vi "Run Framework Configuration.vi"(7 "framework options":T13={"FIFO Options"={"Infinite Timeouts"=FALSE}, "Thread Options"={"Show FP On Call"=TRUE, "Close FP After Call"=TRUE, "Allow Debugging"=FALSE, "Restart On Error"=FALSE}, "Plugin Options"={"Default Components"=TRUE}, "Performance Options"={"Measure Period"=TRUE, "Measure Rx/Tx Duration"=TRUE}}, 9 "target frequency":u32 format="%.0pHz", 10 "components directory":path, 11 "dsf configuration file path":path=path "C:/Users/Admin/Desktop/test.dsf") -> ()   [LabVIEW 2017, in "DSF Core.lvlib"]
uses:
  DSF Core.lvlib
  Classes/Framework/Framework Options.ctl
  Typedefs/DSF FIFO Options.ctl
  Classes/Thread/DSF Thread Options.ctl
  Typedefs/DSF Plugin Options.ctl
  Typedefs/DSF Performance Options.ctl
  Typedefs/DSF Engine Framework Configuration.ctl
  Typedefs/DSF Engine Plugin Configuration.ctl
  Typedefs/DSF Timing Info.ctl
  Typedefs/DSF Engine Plugin Thread Configuration.ctl
  Typedefs/DSF Settings Info.ctl
  Typedefs/DSF Engine Transfer Group Configuration.ctl
  Typedefs/DSF Direction.ctl
  Typedefs/DSF Engine Transfer Configuration.ctl
  Typedefs/DSF Byte Order.ctl
  Typedefs/DSF Engine Channel Configuration.ctl
  Typedefs/DSF Data Type.ctl
  Typedefs/DSF Timeout Behavior.ctl
  <vilib>/NI/Memory Manager/Classes/Pointer/Pointer.lvclass
  <vilib>/NI/Memory Manager/Classes/Pointer/Pointer.lvclass/Pointer.ctl
  <vilib>/Platform/TimedLoop/XDataNode/timing_clust.ctl
  <vilib>/Platform/TimedLoop/XDataNode/nitl_modes.ctl
  <vilib>/Platform/TimedLoop/XDataNode/wakeup.ctl
  <vilib>/NI/Memory Manager/Classes/Pointer/Write U32.vi
  <vilib>/NI/Memory Manager/Classes/Pointer/Read U32.vi
  <vilib>/NI/Memory Manager/Classes/Pointer/Read Bool.vi
  <vilib>/NI/Memory Manager/Classes/Pointer/Write Bool.vi
  <vilib>/NI/Memory Manager/Classes/Pointer/Set Address.vi
  <vilib>/NI/Memory Manager/Classes/Pointer/Set Size.vi
  <vilib>/NI/Memory Manager/Classes/Pointer/Set Internal.vi
  <vilib>/NI/Memory Manager/Classes/Pointer/Check Null Pointer.vi
  <vilib>/NI/Memory Manager/Classes/Pointer/Clear (No Check).vi
  <vilib>/NI/Memory Manager/Classes/Pointer/Check Length.vi
  <vilib>/NI/Memory Manager/Classes/Pointer/Write (No Check).vi
  <vilib>/NI/Memory Manager/Classes/Pointer/Write (No Check) U32.vi
  <vilib>/NI/Memory Manager/Classes/Pointer/Check Move.vi
  <vilib>/NI/Memory Manager/Classes/Pointer/Read (No Check).vi
  <vilib>/NI/Memory Manager/Classes/Pointer/Read (No Check) U32.vi
  <vilib>/NI/Memory Manager/Classes/Pointer/Read (No Check) Bool.vi
  <vilib>/NI/Memory Manager/Classes/Pointer/Write (No Check) Bool.vi
  <vilib>/NI/Memory Manager/Classes/Pointer/Get Internal.vi
  <vilib>/NI/Memory Manager/Classes/Pointer/Errors.vi
  <vilib>/NI/Memory Manager/Classes/Pointer/Zone.vi
  <vilib>/NI/Memory Manager/Classes/Pointer/Null Pointer.vi
  <vilib>/NI/Memory Manager/Classes/Pointer/Check Bounds (Pointer).vi
  <vilib>/NI/Memory Manager/Classes/Pointer/Check Count.vi
  <vilib>/NI/Memory Manager/Classes/Pointer/Check Bounds (Power of 2).vi
  <vilib>/NI/Memory Manager/Classes/Pointer/Create Error.vi
  <vilib>/NI/Memory Manager/Classes/Pointer/Out of Bounds.vi
  <vilib>/NI/Memory Manager/Classes/Pointer/Check Bounds.vi
  <vilib>/NI/Memory Manager/Constants/Constants.vi
  <vilib>/NI/Memory Manager/Constants/Library Name.vi
  <vilib>/NI/Memory Manager/Classes/Pointer/Pointer Error Info.vi
  <vilib>/NI/Memory Manager/Constants/Pointer Class Name.vi
  <vilib>/NI/Memory Manager/Classes/Pointer/Write Pointer Size to Error.vi
  <vilib>/NI/Memory Manager/Classes/Pointer/Check Bounds (Buffer).vi
  <vilib>/NI/Memory Manager/Classes/Pointer/Buffer Underflow.vi
  <vilib>/NI/Memory Manager/VIs/New Error Cluster.vi
  <vilib>/NI/Memory Manager/VIs/New Error Cluster (512B).vi
  <vilib>/NI/Memory Manager/VIs/Set Error Status.vi
  <vilib>/NI/Memory Manager/VIs/Set Error Code.vi
  <vilib>/NI/Memory Manager/VIs/Set Error Source.vi
  <vilib>/NI/Memory Manager/VIs/Write String to Source.vi
  <vilib>/NI/Memory Manager/VIs/Write Numeric to Source.vi
  <vilib>/NI/Memory Manager/VIs/Write Numeric Scalar to Source (Base10 U64).vi
  Classes/Framework/Framework.lvclass
  <vilib>/platform/TimedLoop/XDataNode/XDataNode.xnode
  Classes/Configuration/Configuration Session.lvclass
  <vilib>/Platform/TimedLoop/XDataNode/XDNodeRunTimeDep.lvlib
panel:
  in  "Inline Buffer (null)":refnum<class "Pointer.lvclass">
  out "framework configuration":T1
  out "actual frequency":u32 format="%.0pHz"
  out "iteration":i32
  out "error out":errorcluster
  in  "stop":bool
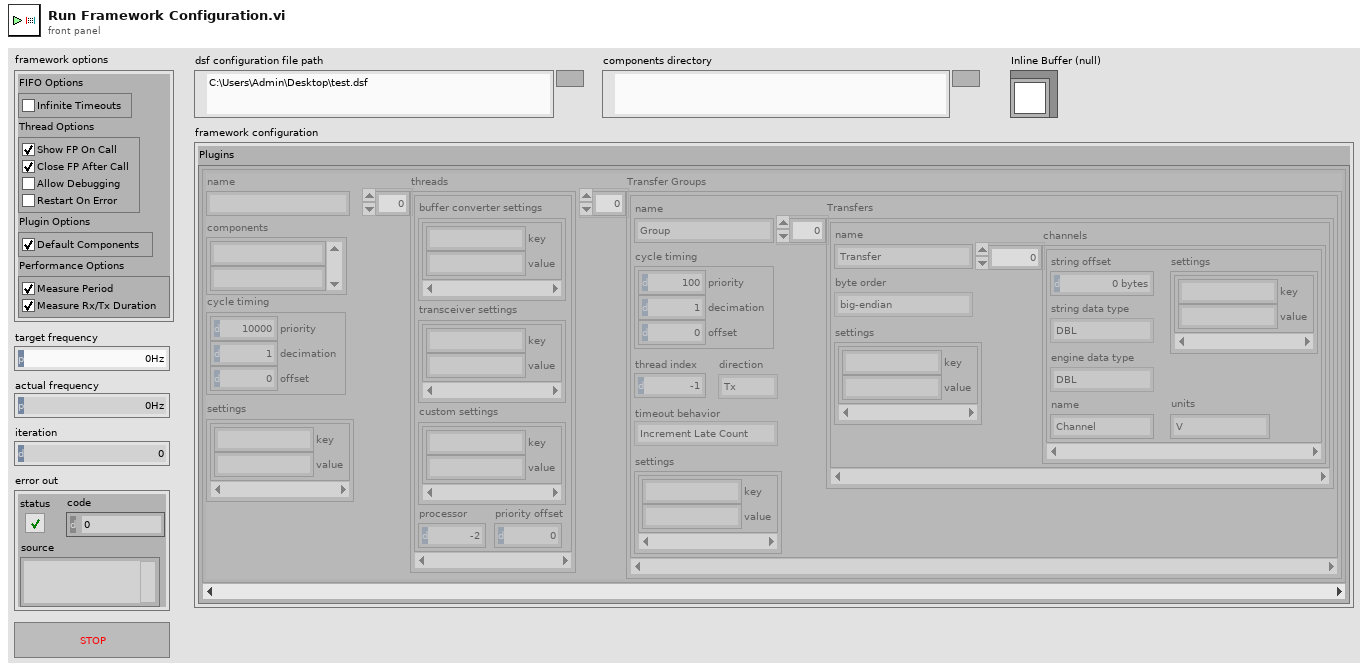
[diagram p1: front panel]
types:
  T1 = typedef "DSF Core.lvlib/DSF Engine Framework Configuration.ctl" = cluster{"Plugins":T2[]}
  T2 = typedef "DSF Core.lvlib/DSF Engine Plugin Configuration.ctl" = cluster{"name":string, "components":string[], "cycle timing":T3, "threads":T4[], "Transfer Groups":T6[], "settings":T5}
  T3 = typedef "DSF Core.lvlib/DSF Timing Info.ctl" = cluster{"priority":u64, "decimation":u64, "offset":u64}
  T4 = typedef "DSF Core.lvlib/DSF Engine Plugin Thread Configuration.ctl" = cluster{"buffer converter settings":T5, "transceiver settings":T5, "custom settings":T5, "processor":i32, "priority offset":i16}
  T5 = typedef "DSF Core.lvlib/DSF Settings Info.ctl" = cluster{"key":string, "value":string}[]
  T6 = typedef "DSF Core.lvlib/DSF Engine Transfer Group Configuration.ctl" = cluster{"name":string, "direction":T7, "cycle timing":T3, "thread index":i32, "settings":T5, "Transfers":T8[], "timeout behavior":T12}
  T7 = typedef "DSF Core.lvlib/DSF Direction.ctl" = enum8{"Tx", "Rx"}
  T8 = typedef "DSF Core.lvlib/DSF Engine Transfer Configuration.ctl" = cluster{"name":string, "byte order":T9, "settings":T5, "channels":T10[]}
  T9 = typedef "DSF Core.lvlib/DSF Byte Order.ctl" = enum8{"big-endian", "little-endian"}
  T10 = typedef "DSF Core.lvlib/DSF Engine Channel Configuration.ctl" = cluster{"string offset":u64, "string data type":T11, "engine data type":T11, "name":string, "settings":T5, "units":string}
  T11 = typedef "DSF Core.lvlib/DSF Data Type.ctl" = enum8{"Bool", "SGL", "DBL", "I8", "I16", "I32", "I64", "U8", "U16", "U32", "U64"}
  T12 = typedef "DSF Core.lvlib/DSF Timeout Behavior.ctl" = enum8{"Increment Late Count", "Throw Error"}
  T13 = typedef "DSF Core.lvlib/Framework.lvclass/Framework Options.ctl" = cluster{"FIFO Options":T14, "Thread Options":T15, "Plugin Options":T16, "Performance Options":T17}
  T14 = typedef "DSF Core.lvlib/DSF FIFO Options.ctl" = cluster{"Infinite Timeouts":bool}
  T15 = typedef "DSF Core.lvlib/DSF Thread Options.ctl" = cluster{"Show FP On Call":bool, "Close FP After Call":bool, "Allow Debugging":bool, "Restart On Error":bool}
  T16 = typedef "DSF Core.lvlib/DSF Plugin Options.ctl" = cluster{"Default Components":bool}
  T17 = typedef "DSF Core.lvlib/DSF Performance Options.ctl" = cluster{"Measure Period":bool, "Measure Rx/Tx Duration":bool}
  T18 = typedef "XDNodeRunTimeDep.lvlib/timing_clust.ctl" = cluster{"Expected End [f-1]":u64, "Actual End [f-1]":u64, "Finished Late? [f-1]":bool, "Expected End [i-1]":u64, "Actual End [i-1]":u64, "Finished Late? [i-1]":bool, "Expected Start [i]":u64, "Actual Start [i]":u64, "Expected Start [f]":u64, "Actual Start [f]":u64, "Source Name":string, "Structure Name":string, "Period":i64, "Deadline":i64, "Offset":i64, "Start":i64, "Priority":i32, "Timeout":i32, "Mode":T19, "Wakeup Reason":T20, "Error":errorcluster, "Source Type":string, "Secondary Source Type":string, "Global End Time":u64, "Global Start Time":u64, "Frame Duration":u64, "Iteration Duration":u64, "Assigned CPU":i32, "I/O Scan Engine Mode":u32}
  T19 = typedef "XDNodeRunTimeDep.lvlib/nitl_modes.ctl" = enum32{"No Change", "Process missed periods, maintain original phase", "Discard missed periods, maintain original phase", "Process missed periods, ignore original phase", "Discard missed periods, ignore original phase"}
  T20 = typedef "XDNodeRunTimeDep.lvlib/wakeup.ctl" = enum32{"Normal", "Aborted", "Asynchronous wakeup", "Timing source error", "Timed loop error", "Timeout"}
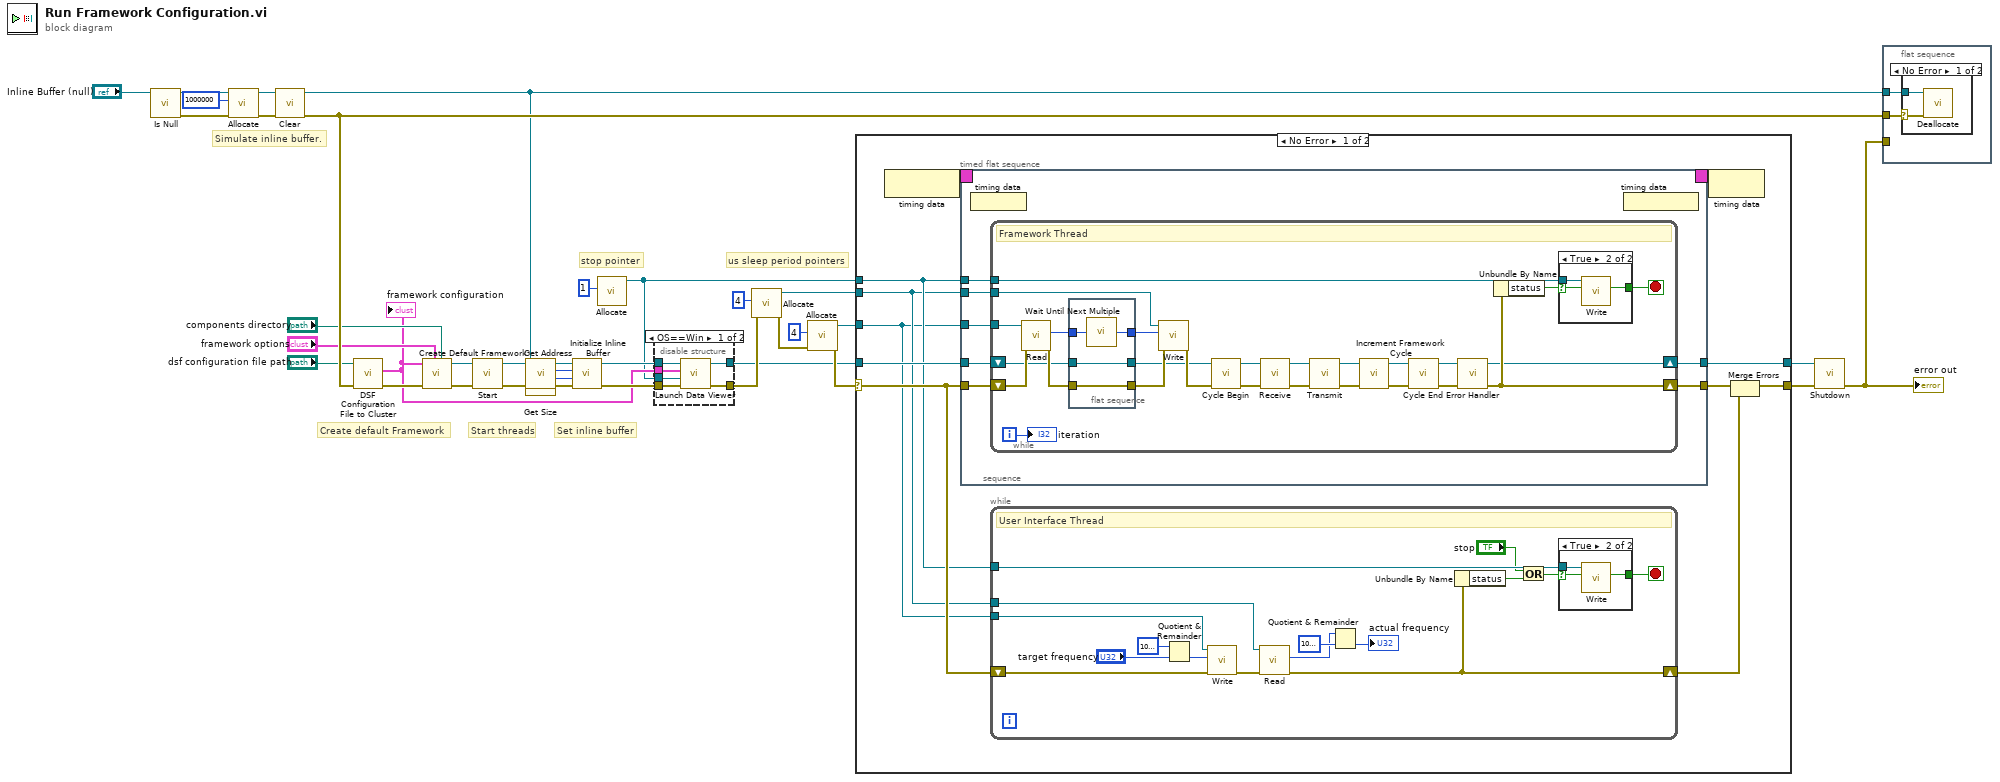
[diagram p0: block diagram]
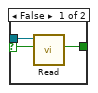
[diagram p4: hidden frame]
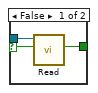
[diagram p5: hidden frame]
diagram:
  # "us sleep period pointers"
  # "stop pointer"
  # "Set inline buffer"
  # "Start threads"
  # "Create default Framework"
  # "Simulate inline buffer."
  n1 = call <vilib>:"Is Null.vi"("Pointer in"="Inline Buffer (null)") -> ("error out"=w1:errorcluster, "Pointer out"=w2:refnum<class "Pointer.lvclass">)  [unwired: 8 in, 1 out]
  n2 = call <vilib>:"Allocate.vi"("error in (no error)"=w1, "size"=u64 1000000, "Pointer type"=w2) -> ("error out"=w29:errorcluster, "Pointer out"=w26:refnum<class "Pointer.lvclass">)  [unwired: 7 in]
  n3 = call <vilib>:"Clear.vi"("error in (no error)"=w29, "Pointer in"=w26) -> ("error out"=w34:errorcluster, "Pointer out"=w14:refnum<class "Pointer.lvclass">)  [unwired: 8 in]
  n4 = call "DSF Configuration File to Cluster.vi"("error in (no error)"=w34, "dsf configuration file path"="dsf configuration file path") -> ("error out"=w25:errorcluster, "framework configuration out"=w13:T1)  [unwired: 7 in, 1 out]
  "framework configuration" <- w13
  n5 = call "Create Default Framework.vi"("components directory (default)"="components directory", "framework options"="framework options", "error in (no error)"=w25, "framework configuration"=w13) -> ("error out"=w17:errorcluster, "Framework"=w23:refnum<class "Framework.lvclass">)  [unwired: 6 in]
  n6 = call-dynamic "Start.vi"("error in (no error)"=w17, "Framework in"=w23) -> ("error out"=w22:errorcluster, "Framework out"=w33:refnum<class "Framework.lvclass">)  [unwired: 8 in]
  n7 = call <vilib>:"Get Address.vi"("Pointer in"=w14) -> ("address"=w27:u64)  [unwired: 9 in, 1 out]
  n8 = call <vilib>:"Get Size.vi"("Pointer in"=w14) -> ("size"=w28:u64)  [unwired: 9 in, 1 out]
  n9 = call "Initialize Inline Buffer.vi"("error in (no error)"=w22, "size"=w28, "address"=w27, "Framework in"=w33) -> ("error out"=w20:errorcluster, "Framework out"=w21:refnum<class "Framework.lvclass">)  [unwired: 6 in]
  n10 = call <vilib>:"Allocate.vi"("size"=u64 1) -> ("Pointer out"=w11:refnum<class "Pointer.lvclass">)  [unwired: 9 in, 1 out]
  n11 = disable-structure shown="OS==Win" {
    disable-tunnel: [w40 w42] -> w4
    disable-tunnel: [w39 w41] -> w5
    disable-tunnel: w21 -> [w38 w42]
    disable-tunnel: w20 -> [w37 w41]
    disable-tunnel: w13 -> [w36 _]
    disable-tunnel: w11 -> [w35 _]
    frame condition #0 (active) {
      n12 = call "Launch Data Viewer.vi"("error in (no error)"=w37, "Stop Pointer"=w35, "Framework Configuration"=w36, "Framework in"=w38) -> ("error out"=w39:errorcluster, "Framework out"=w40:refnum<class "Framework.lvclass">)  [unwired: 6 in]
    }
    frame condition #1 {
    }
  }
  n13 = call <vilib>:"Allocate.vi"("error in (no error)"=w5, "size"=u64 4) -> ("error out"=w6:errorcluster, "Pointer out"=w7:refnum<class "Pointer.lvclass">)  [unwired: 8 in]
  n14 = call <vilib>:"Allocate.vi"("error in (no error)"=w6, "size"=u64 4) -> ("error out"=w9:errorcluster, "Pointer out"=w10:refnum<class "Pointer.lvclass">)  [unwired: 8 in]
  n15 = case shown="No Error" w9 {
    selector: w9 -> [w53 w130]
    tunnel: [w44 w130] -> w32
    tunnel: w4 -> [w52 w131]
    tunnel: [w51 w131] -> w31
    tunnel: w11 -> [w48 _]
    tunnel: w10 -> [w46 _]
    tunnel: w7 -> [w47 _]
    frame No Error {
      n16 = node-c288() -> (w50:T18)
      n17 = timed-sequence {
        timing: w50 -> [_]
        timing-out: [_] -> w49
        tunnel: w52 -> [w82]
        tunnel: w53 -> [w81]
        tunnel: [w80] -> w51
        tunnel: [w79] -> w45
        tunnel: w48 -> [w78]
        tunnel: w46 -> [w77]
        tunnel: w47 -> [w76]
        n18 = timed-flat-sequence {
          tunnel: w82 -> [w89]
          tunnel: w81 -> [w88]
          tunnel: [w87] -> w80
          tunnel: [w86] -> w79
          tunnel: w78 -> [w85]
          tunnel: w77 -> [w84]
          tunnel: w76 -> [w83]
          n19 = node-c288() -> ()  [unwired: 1 in]
          n20 = while {
            shift-right: [w101] -> w87
            shift-left: w89 -> [w102]
            tunnel: w85 -> [w113]
            shift-right: [w107] -> w86
            shift-left: w88 -> [w104]
            tunnel: w84 -> [w105]
            tunnel: w83 -> [w96]
            i -> [w109]
            stop <- w112 stop-if-true
            # "Framework Thread"
            n21 = call-poly <vilib>:"Read.vi"("error in (no error)"=w104, "Pointer in"=w105) -> ("error out"=w103:errorcluster, "value out"=w106:u32)  [unwired: 6 in, 2 out]
            n22 = flat-sequence {
              tunnel: w102 -> [w119]
              tunnel: w103 -> [w118]
              tunnel: [w119] -> w97
              tunnel: [w118] -> w98
              tunnel: w106 -> [w117]
              tunnel: [w116] -> w100
              frame #0 {
                n23 = call "Wait Until Next Multiple"("Count(uSec)"=w117) -> ("Tick Count(uSec)"=w116:u32)
              }
            }
            n24 = call-poly <vilib>:"Write.vi"("error in (no error)"=w98, "value"=w100, "Pointer in"=w96) -> ("error out"=w99:errorcluster)  [unwired: 5 in, 3 out]
            n25 = call "Cycle Begin.vi"("error in (no error)"=w99, "Framework in"=w97) -> ("error out"=w110:errorcluster, "Framework out"=w111:refnum<class "Framework.lvclass">)  [unwired: 8 in]
            n26 = call "Receive.vi"("error in (no error)"=w110, "Framework in"=w111) -> ("error out"=w115:errorcluster, "Framework out"=w114:refnum<class "Framework.lvclass">)  [unwired: 8 in]
            n27 = call "Transmit.vi"("error in (no error)"=w115, "Framework in"=w114) -> ("error out"=w95:errorcluster, "Framework out"=w94:refnum<class "Framework.lvclass">)  [unwired: 8 in]
            n28 = call "Increment Framework Cycle.vi"("error in (no error)"=w95, "Framework in"=w94) -> ("error out"=w92:errorcluster, "Framework out"=w93:refnum<class "Framework.lvclass">)  [unwired: 8 in]
            n29 = call "Cycle End.vi"("error in (no error)"=w92, "Framework in"=w93) -> ("error out"=w91:errorcluster, "Framework out"=w90:refnum<class "Framework.lvclass">)  [unwired: 8 in]
            n30 = call "Error Handler.vi"("error in (no error)"=w91, "Framework in"=w90) -> ("error out"=w107:errorcluster, "Framework out"=w101:refnum<class "Framework.lvclass">)  [unwired: 8 in]
            n31 = Unbundle By Name(w107) -> ("status"=w108:bool)
            n32 = case shown="True" w108 {
              selector: w108 -> [w121 w124]
              tunnel: w113 -> [w122 w125]
              tunnel: [w120 w123] -> w112
              frame False {
                n33 = call-poly <vilib>:"Read.vi"("value in"=w121, "Pointer in"=w122) -> ("value out"=w120:bool)  [unwired: 6 in, 3 out]
              }
              frame True {
                n34 = call-poly <vilib>:"Write.vi"("value"=w124, "Pointer in"=w125) -> ("value"=w123:bool)  [unwired: 6 in, 3 out]
              }
            }
            "iteration" <- w109
          }
          n35 = node-c288() -> ()  [unwired: 1 out]
        }
      }
      n36 = while {
        tunnel: w48 -> [w69]
        shift-right: [w60] -> w43
        shift-left: w53 -> [w64]
        tunnel: w46 -> [w59]
        tunnel: w47 -> [w54]
        stop <- w68 stop-if-true
        # "User Interface Thread"
        n37 = Quotient & Remainder(x=u32 1000000 ("y"), y="target frequency") -> (floor(x/y)=w55:u32)  [unwired: 1 out]
        n38 = call-poly <vilib>:"Write.vi"("error in (no error)"=w64, "value"=w55, "Pointer in"=w59) -> ("error out"=w61:errorcluster)  [unwired: 5 in, 3 out]
        n39 = call-poly <vilib>:"Read.vi"("error in (no error)"=w61, "Pointer in"=w54) -> ("error out"=w60:errorcluster, "value out"=w56:u32)  [unwired: 6 in, 2 out]
        n40 = Quotient & Remainder(x=w56, y=u32 1000000) -> (floor(x/y)=→"actual frequency":u32)  [unwired: 1 out]
        n41 = Unbundle By Name(w60) -> ("status"=w66:bool)
        n42 = Or(x="stop", y=w66) -> (x .or. y?=w67:bool)
        n43 = case shown="True" w67 {
          selector: w67 -> [w71 w74]
          tunnel: w69 -> [w72 w75]
          tunnel: [w70 w73] -> w68
          frame False {
            n44 = call-poly <vilib>:"Read.vi"("value in"=w71, "Pointer in"=w72) -> ("value out"=w70:bool)  [unwired: 6 in, 3 out]
          }
          frame True {
            n45 = call-poly <vilib>:"Write.vi"("value"=w74, "Pointer in"=w75) -> ("value"=w73:bool)  [unwired: 6 in, 3 out]
          }
        }
      }
      n46 = node-c288(w49) -> ()
      n47 = Merge Errors(w45, w43) -> (w44:errorcluster)
    }
    frame Error {
    }
  }
  n48 = call-dynamic "Shutdown.vi"("error in (no error)"=w32, "Framework in"=w31) -> ("error out"=w15:errorcluster)  [unwired: 8 in, 1 out]
  "error out" <- w15
  n49 = flat-sequence {
    tunnel: w14 -> [w133]
    tunnel: w15 -> [_]
    tunnel: w34 -> [w132]
    frame #0 {
      n50 = case shown="No Error" w132 {
        selector: w132 -> [w134 _]
        tunnel: w133 -> [w135 _]
        frame No Error {
          n51 = call <vilib>:"Deallocate.vi"("error in (no error)"=w134, "Pointer"=w135) -> ()  [unwired: 8 in, 2 out]
        }
        frame Error {
        }
      }
    }
  }
